vi "S7_Build_Message.vi"(9 "Write Data":i32 format="%08x", 10 "Parameters":u8[](array[numeric]) format="%02x", 11 "Exchange PDU":bool) -> (3 "S7 Ethernet Data":u8[](array[numeric]) format="%02x")   [LabVIEW 2017, in "S7 TCP.lvlib"]
uses:
  S7 TCP.lvlib
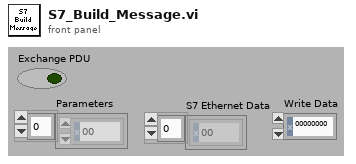
[diagram p1: front panel]
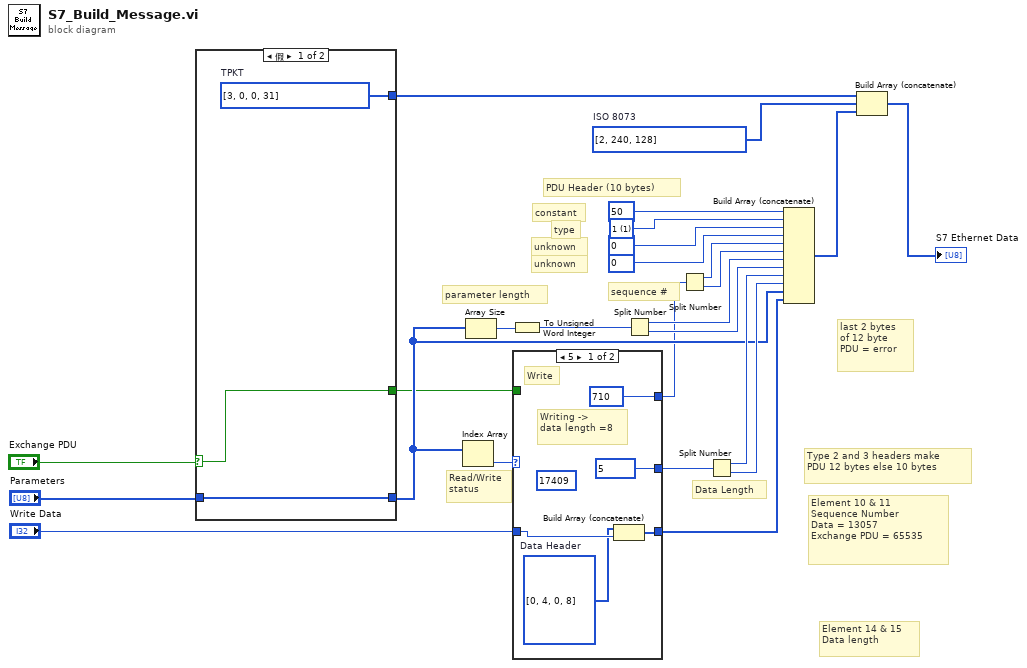
[diagram p0: block diagram]
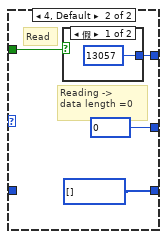
[diagram p2: hidden frame]
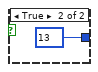
[diagram p3: hidden frame]
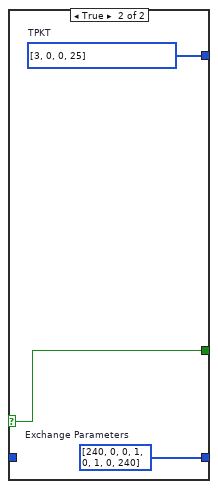
[diagram p4: hidden frame]
diagram:
  w5 = u8[] [2, 240, 128]  # ISO 8073
  w22 = u8 1 items=["1"=1, "2"=2, "3"=3, "7"=7]
  # "parameter length"
  # "Data Length"
  # "Read/Write status"
  # "sequence #"
  # "Element 10 & 11\nSequence Number\nData = 13057\nExchange PDU = 65535"
  # "Element 14 & 15\nData length"
  # "last 2 bytes\nof 12 byte\nPDU = error"
  # "Type 2 and 3 headers make\nPDU 12 bytes else 10 bytes"
  # "constant"
  # "type"
  # "unknown"
  # "unknown"
  # "PDU Header (10 bytes)"
  n1 = case shown="假" "Exchange PDU" {
    selector: "Exchange PDU" -> [w27 w30]
    tunnel: [w28 w31] -> w8
    tunnel: "Parameters" -> [w28 _]
    tunnel: [w27 w30] -> w2
    tunnel: [w26 w29] -> w1
    frame False {
      w26 = u8[] [3, 0, 0, 31]  # TPKT
    }
    frame True {
      w29 = u8[] [3, 0, 0, 25]  # TPKT
      w31 = u8[] [240, 0, 0, 1, 0, 1, 0, 240]  # Exchange Parameters
    }
  }
  n2 = Index Array(array=w8) -> (element=w19:u8)  [unwired: 1 in]
  n3 = Array Size(array=w8) -> (size(s)=w10:i32)
  n4 = To Unsigned Word Integer(number=w10) -> (unsigned 16bit integer=w9:u16)
  n5 = case shown="5" w19 {
    tunnel: [u16 5 ("DLE") u16 0 ("DLE")] -> w15
    tunnel: "Write Data" -> [w35 _]
    tunnel: [w34 u8[] []] -> w13
    tunnel: [u16 710 ("DLE") w38] -> w6
    tunnel: w2 -> [_ w37]
    frame 5 {
      (unwired) u16 17409 ("DLE")
      w33 = u8[] [0, 4, 0, 8]  # Data Header
      # "Write"
      # "Writing ->\ndata length =8"
      n6 = Build Array (concatenate)(w33, w35) -> (w34:i32[])
    }
    frame 4, Default {
      # "Read"
      # "Reading ->\ndata length =0"
      n7 = case shown="假" w37 {
        tunnel: [u16 13057 ("DLE") u16 13 ("DLE")] -> w38
        frame False {
        }
        frame True {
        }
      }
    }
  }
  n8 = Split Number(x=w9) -> (hi(x)=w25:u8, lo(x)=w18:u8)
  n9 = Split Number(x=w6) -> (hi(x)=w12:u8, lo(x)=w11:u8)
  n10 = Split Number(x=w15) -> (hi(x)=w17:u8, lo(x)=w16:u8)
  n11 = Build Array (concatenate)(u8 50 ("DLE"), w22, u8 0 ("DLE"), u8 0 ("DLE"), w12, w11, w25, w18, w17, w16, w8, w13) -> (w4:i32[])
  n12 = Build Array (concatenate)(w1, w5, w4) -> (→"S7 Ethernet Data":i32[])
